vi "rotate if needed.vi"(8 "error in":errorcluster, 9 "Check?":bool, 10 "LogRotate":refnum<class "LogRotate.lvclass">, 11 "tdms ref in":refnum<k34>) -> (0 "error out":errorcluster, 2 "rotated?":bool, 3 "tdms ref out":refnum<k34>)   [LabVIEW 2013, in "TDMS datalogger runtime.lvclass"]
uses:
  TDMS datalogger runtime.lvclass
  <vilib>/NI/LogRotate/LogRotate.lvclass
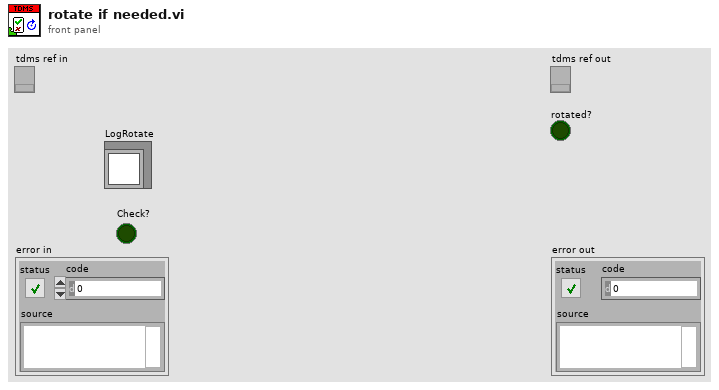
[diagram p1: front panel]
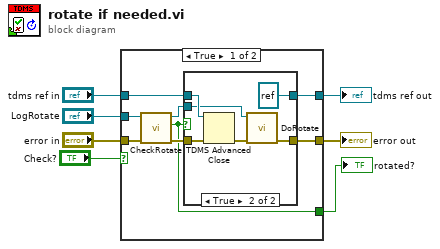
[diagram p0: block diagram]
diagram:
  n1 = case shown="True" "Check?" {
    selector: "Check?" -> [_ w24]
    tunnel: "LogRotate" -> [w15 _]
    tunnel: "error in" -> [w14 w26]
    tunnel: [w9 w26] -> w6
    tunnel: "tdms ref in" -> [w13 w25]
    tunnel: [w12 w25] -> w4
    tunnel: [w8 w24] -> w1
    frame True {
      n2 = call <vilib>:"CheckRotate.vi"("error in (no error)"=w14, "LogRotate in"=w15) -> ("error out"=w10:errorcluster, "Rotate?"=w8:bool, "LogRotate out"=w11:refnum<class "LogRotate.lvclass">)  [unwired: 7 in]
      n3 = case shown="True" w8 {
        tunnel: w13 -> [w17 w23]
        tunnel: [w17 refnum<k34> refnum ("tdms ref in")] -> w12
        tunnel: w11 -> [_ w22]
        tunnel: w10 -> [w16 w19]
        tunnel: [w16 w18] -> w9
        frame False {
        }
        frame True {
          n4 = TDMS Advanced Close(8:w19, 11:w23) -> (0:w21:errorcluster)  [unwired: 2 in, 1 out]
          n5 = call <vilib>:"DoRotate.vi"("error in (no error)"=w21, "LogRotate in"=w22) -> ("error out"=w18:errorcluster)  [unwired: 8 in, 1 out]
        }
      }
    }
    frame False {
    }
  }
  "error out" <- w6
  "tdms ref out" <- w4
  "rotated?" <- w1
